vi "Myrio_12.vi"   [LabVIEW 2012]
uses:
  SubVIs/LVPresent_Globals.vi
panel:
  # "Scripting"
  # "In Botspeak you can use the scripting library to write programs that the myRIO can run without being tethered to the computer."
  # "This is a program that will blink LED0 once. Try detatching it from the computer; it will still run."
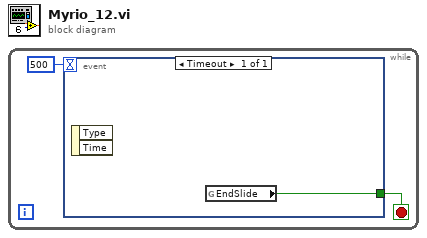
[diagram p0: block diagram]
diagram:
  n1 = while {
    stop <- w2 stop-if-true
    n2 = event shown="[0] Timeout" {
      selector: _ -> [_]
      dyn-events: _ -> [_]
      timeout: 500 -> [_]
      tunnel: [w3] -> w2
      event Timeout {
        n3 = event-data() -> ()  [unwired: 1 in, 2 out]
        n4 = global read "LVPresent_Globals.vi" "EndSlide"() -> (w3:bool)
      }
    }
  }
